vi "Create XY Controller.vi"(8 "error in (no error)":errorcluster, 10 "Y-Axis":refnum<class "iMotion Controller.lvclass">, 11 "X-Axis":refnum<class "iMotion Controller.lvclass">) -> (0 "error out":errorcluster, 3 "XY Stage Controller out":refnum<class "XY Stage Controller.lvclass">)   [LabVIEW 2022 SP3, in "XY Stage Controller.lvclass"]
uses:
  XY Stage Controller.lvclass
  Axis Objects/iMotion Controller/iMotion Controller.lvclass
  XY Stage Process/XY Stage Process/XY Stage Process/XY Stage Process.lvclass
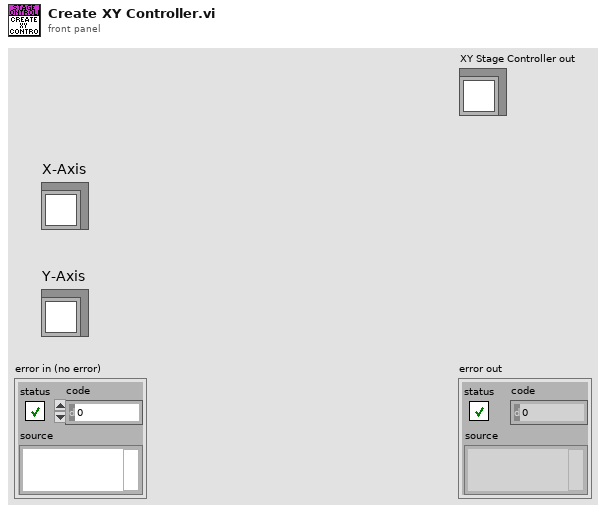
[diagram p1: front panel]
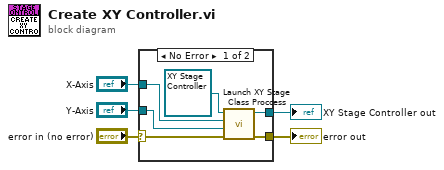
[diagram p0: block diagram]
diagram:
  n1 = case shown="No Error" "error in (no error)" {
    selector: "error in (no error)" -> [w9 w12]
    tunnel: [w8 w12] -> w4
    tunnel: [w10 _] -> w3
    tunnel: "Y-Axis" -> [w6 _]
    tunnel: "X-Axis" -> [w7 _]
    frame No Error {
      n2 = call "Launch XY Stage Class Proccess.vi"("error in (no error)"=w9, "Y Stage"=w6, "X Stage"=w7, "XY Stage Controller in"=refnum<class "XY Stage Controller.lvclass"> refnum) -> ("error out"=w8:errorcluster, "XY Stage Controller out"=w10:refnum<class "XY Stage Controller.lvclass">)  [unwired: 6 in]
    }
    frame Error {
    }
  }
  "error out" <- w4
  "XY Stage Controller out" <- w3
